vi "Timed Loop Time.vi"(8 "error in (no error)":errorcluster, 10 "ET since start (s)":dbl, 11 "State in":T1={"State"=enum."Idle", "Start Time"=timestamp(0 s since 1904-01-01), "Current Time"=timestamp(0 s since 1904-01-01), "First Iteration"=FALSE, "Process Name"="", "Output Error"=FALSE, "Log Started"=FALSE, "Cycle Period"=50.0, "Configuration"={"Valve Settings"={"D-O Settings"={"DAQmx Task Name"="", "Output Channel"=0, "Output Channel Names"=[]}, "VICI Electronic Actuator"={"VISA resource name"="", "Mode"=enum."Two Positions With Stops", "Simulated"=FALSE}}, "Valve Type"=enum."Digital Output Valve", "Time On (Sec)"=0.0, "Time Off (Sec)"=0.0, "Run?"=FALSE}, "Data"={"D-O State"=enum."Off"}} {"Configuration"."Valve Settings"."D-O Settings"."Output Channel" items=["Choose a Channel"]}) -> (0 "error out":errorcluster, 3 "State out":T1={"State"=enum."Idle", "Start Time"=timestamp(0 s since 1904-01-01), "Current Time"=timestamp(0 s since 1904-01-01), "First Iteration"=FALSE, "Process Name"="", "Output Error"=FALSE, "Log Started"=FALSE, "Cycle Period"=50.0, "Configuration"={"Valve Settings"={"D-O Settings"={"DAQmx Task Name"="", "Output Channel"=0, "Output Channel Names"=[]}, "VICI Electronic Actuator"={"VISA resource name"="", "Mode"=enum."Two Positions With Stops", "Simulated"=FALSE}}, "Valve Type"=enum."Digital Output Valve", "Time On (Sec)"=0.0, "Time Off (Sec)"=0.0, "Run?"=FALSE}, "Data"={"D-O State"=enum."Off"}} {"Configuration"."Valve Settings"."D-O Settings"."Output Channel" items=["Choose a Channel"]})   [LabVIEW 2018, in "D-O Module.lvlib" / "D-O Module Engine.lvlib"]
uses:
  D-O Module Engine.lvlib
  State Cluster.ctl
  State Enum.ctl
  Valve Clusters.ctl
  D-O Module Settings Cluster.ctl
  D-O Device Settings Cluster.ctl
  VICI Electronic Actuator/VICI Electronic Actuator Settings.ctl
  D-O Module.lvlib
  DIO Valve/VICI Electronic Actuator.lvlib
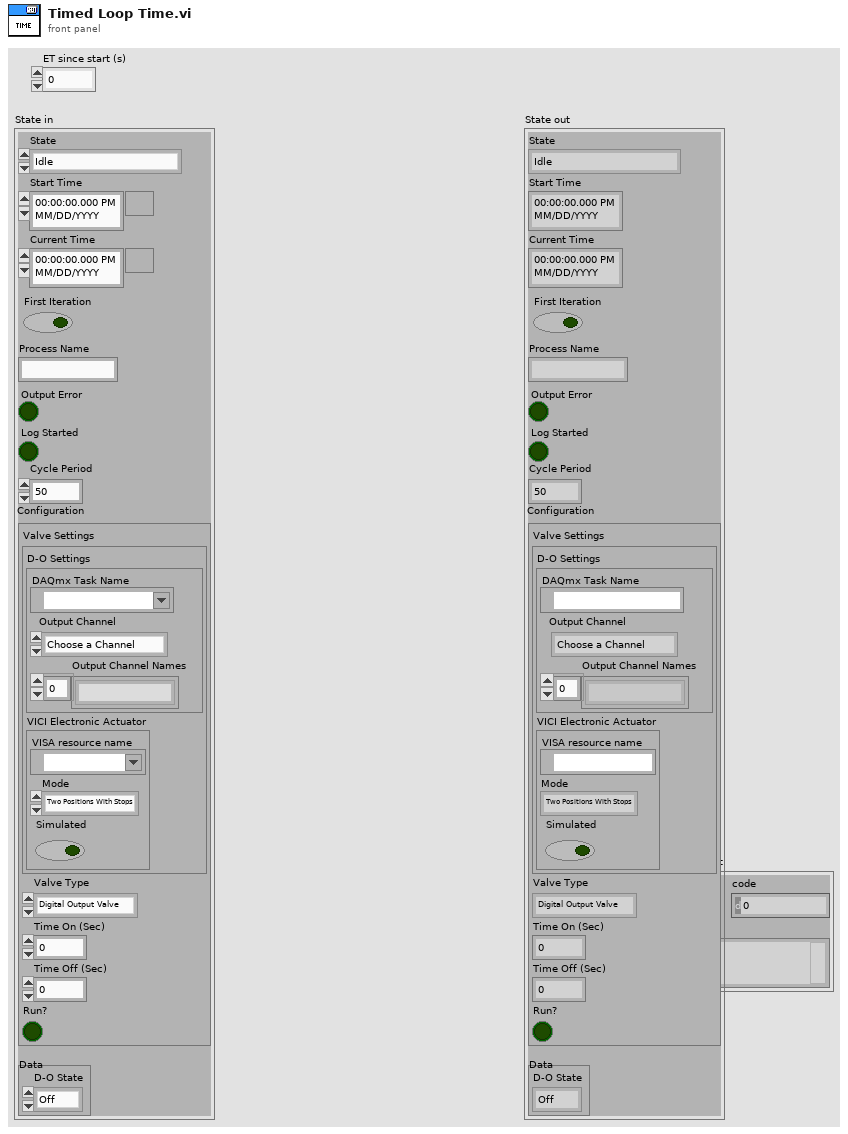
[diagram p1: front panel]
types:
  T1 = typedef "D-O Module.lvlib/D-O Module Engine.lvlib/State Cluster.ctl" = cluster{"State":T2, "Start Time":timestamp, "Current Time":timestamp, "First Iteration":bool, "Process Name":string, "Output Error":bool, "Log Started":bool, "Cycle Period":dbl, "Configuration":T3, "Data":cluster{"D-O State":enum16{"Off", "On", "Not Initialized"}}}
  T2 = typedef "D-O Module.lvlib/D-O Module Engine.lvlib/State Enum.ctl" = enum16{"Measuring", "Idle", "Paused"}
  T3 = typedef "D-O Module.lvlib/Valve Clusters.ctl" = cluster{"Valve Settings":T4, "Valve Type":enum16{"Default", "Digital Output Valve", "VICI Electronic Actuator"}, "Time On (Sec)":dbl, "Time Off (Sec)":dbl, "Run?":bool}
  T4 = typedef "D-O Module.lvlib/D-O Module Settings Cluster.ctl" = cluster{"D-O Settings":T5, "VICI Electronic Actuator":T6}
  T5 = typedef "D-O Module.lvlib/D-O Device Settings Cluster.ctl" = cluster{"DAQmx Task Name":refnum<k21>, "Output Channel":u16, "Output Channel Names":string[]}
  T6 = typedef "VICI Electronic Actuator.lvlib/VICI Electronic Actuator Settings.ctl" = cluster{"VISA resource name":refnum<visa-resource-name>, "Mode":enum16{"Two Positions With Stops", "Two Positions Without Stops", "Mutiposition"}, "Simulated":bool}
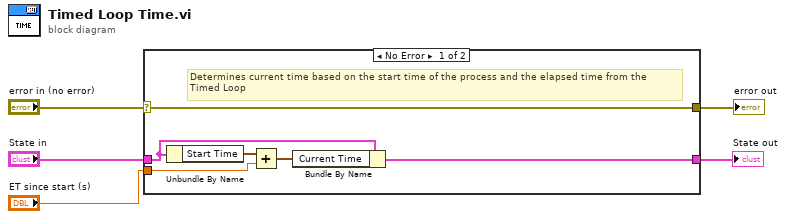
[diagram p0: block diagram]
diagram:
  n1 = case shown="No Error" "error in (no error)" {
    selector: "error in (no error)" -> [w6 w13]
    tunnel: [w6 w13] -> w4
    tunnel: "State in" -> [w11 w12]
    tunnel: [w10 w12] -> w2
    tunnel: "ET since start (s)" -> [w8 _]
    frame No Error {
      # "Determines current time based on the start time of the process and the elapsed time from the\nTimed Loop"
      n2 = Unbundle By Name(w11) -> ("Start Time"=w9:timestamp)
      n3 = Add(x=w9, y=w8) -> (x+y=w7:timestamp)
      n4 = Bundle By Name(cluster=w11, "Current Time"=w7) -> (w10:T1)
    }
    frame Error {
    }
  }
  "error out" <- w4
  "State out" <- w2
